vi "Transmitter.vi"   [LabVIEW 2016]
uses:
  Global Variable.vi
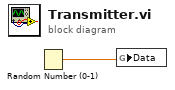
[diagram p0: block diagram]
diagram:
  n1 = Random Number (0-1)() -> (number: 0 to 1=w1:dbl)
  n2 = global write "Global Variable.vi" "Data"(w1) -> ()
